vi "MAVLink Message State Machine.vi"(8 "Error In":errorcluster, 11 "Incoming Bytes":u8) -> (0 "Error Out":errorcluster, 1 "Aircraft ID":u8, 2 "Message":string, 3 "Message Complete":bool)   [LabVIEW 2014]
uses:
  CRC/MAVLink CRC v2 Check.vi
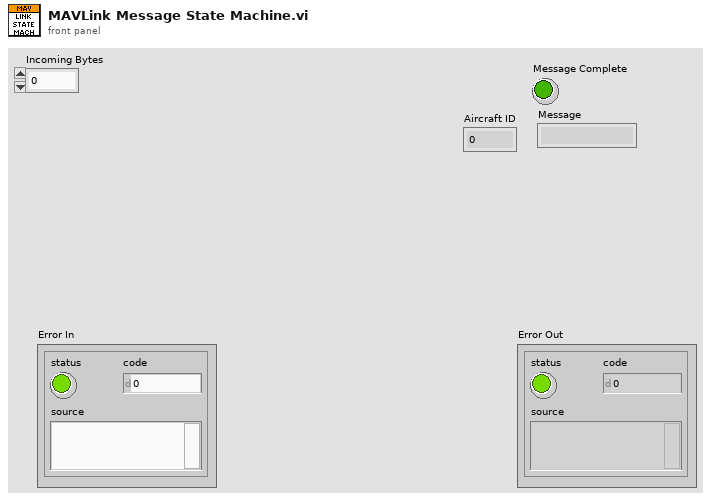
[diagram p1: front panel]
types:
  T1 = enum16{"Waiting For Start Byte", "Calculate Message Size", "Build Message"}
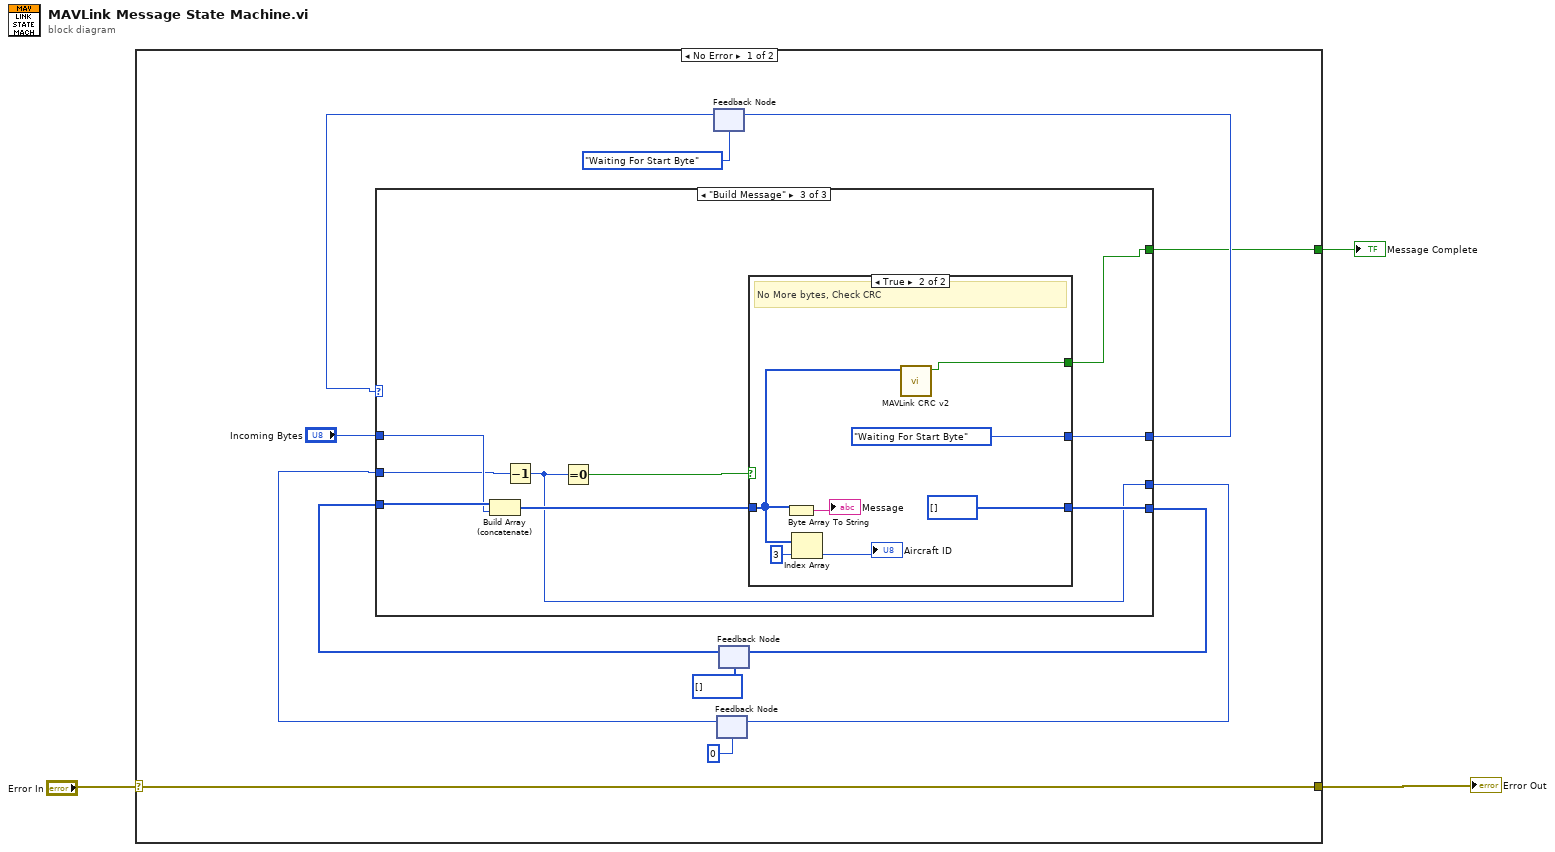
[diagram p0: block diagram]
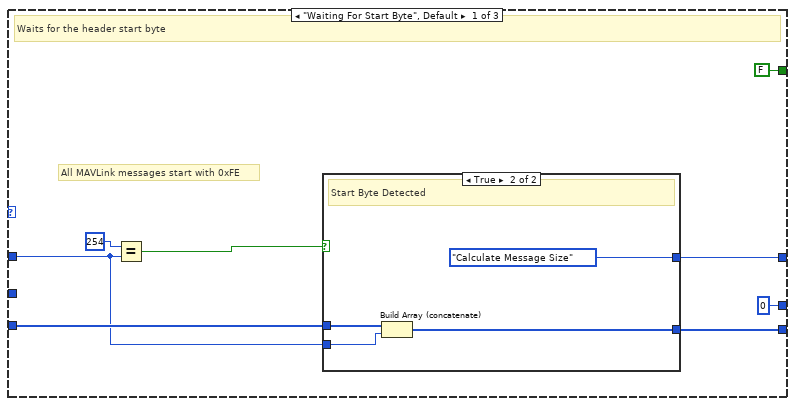
[diagram p2: hidden frame]
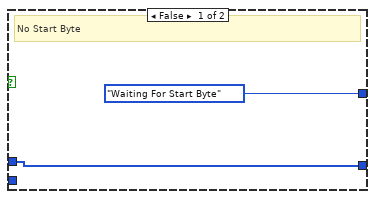
[diagram p3: hidden frame]
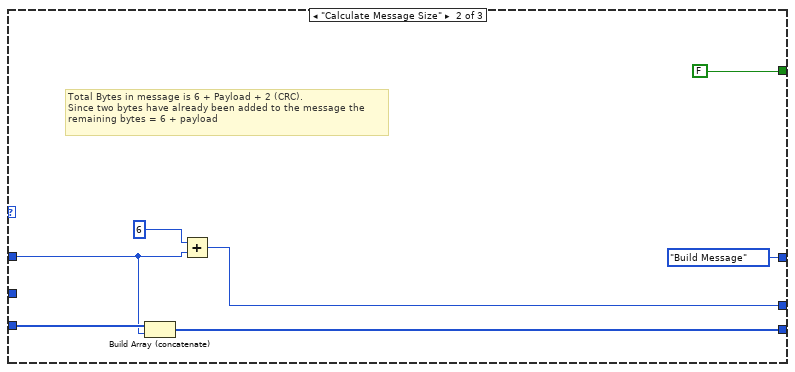
[diagram p4: hidden frame]
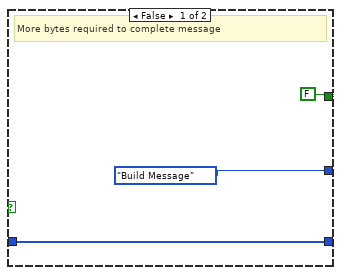
[diagram p5: hidden frame]
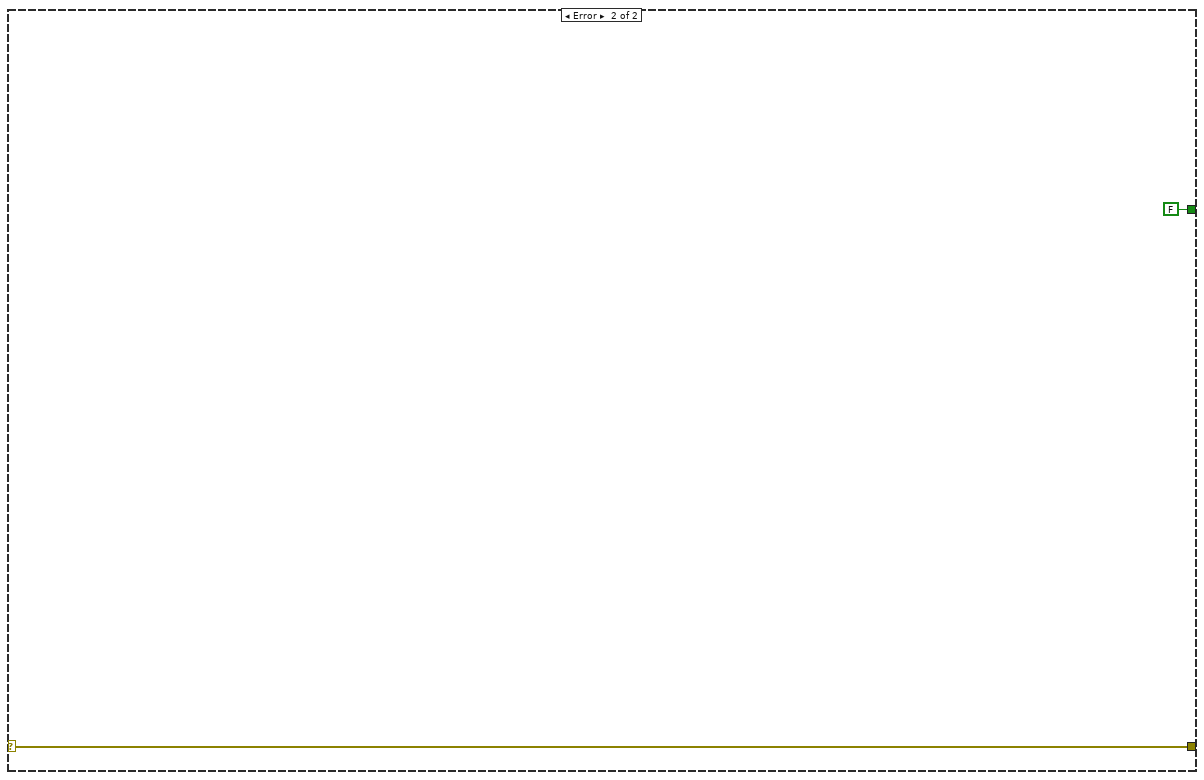
[diagram p6: hidden frame]
diagram:
  n1 = case shown="No Error" "Error In" {
    selector: "Error In" -> [w4 w57]
    tunnel: [w5 FALSE ("CRC good")] -> w3
    tunnel: [w4 w57] -> w1
    frame No Error {
      n2 = feedback #1(T1."Waiting For Start Byte" ("Message States")) -> (w14:T1)
      n3 = feedback #2(u8 0 ("x")) -> (w7:u8)
      n4 = feedback #3(u8[] []) -> (w12:u8[])
      n5 = case shown="\"Build Message\"" w14 {
        tunnel: w12 -> [w21 w34 w45]
        tunnel: "Incoming Bytes" -> [w20 w33 w44]
        tunnel: [w19 w32 w41] -> w10
        tunnel: [w18 T1."Build Message" ("Message States") w40] -> w9
        tunnel: w7 -> [_ _ w43]
        tunnel: [u8 0 w31 w39] -> w6
        tunnel: [FALSE FALSE w37] -> w5
        frame "Waiting For Start Byte", Default {
          # "All MAVLink messages start with 0xFE"
          # "Waits for the header start byte"
          n6 = Equal?(x=u8 254, y=w20) -> (x = y?=w22:bool)
          n7 = case shown="True" w22 {
            tunnel: w21 -> [w25 w29]
            tunnel: w20 -> [_ w28]
            tunnel: [w25 w27] -> w19
            tunnel: [T1."Waiting For Start Byte" ("Message States") T1."Calculate Message Size" ("Message States")] -> w18
            frame False {
              # "No Start Byte"
            }
            frame True {
              # "Start Byte Detected"
              n8 = Build Array (concatenate)(w29, w28) -> (w27:u8[])
            }
          }
        }
        frame "Calculate Message Size" {
          # "Total Bytes in message is 6 + Payload + 2 (CRC).\nSince two bytes have already been added to the message the\nremaining bytes = 6 + payload"
          n9 = Build Array (concatenate)(w34, w33) -> (w32:u8[])
          n10 = Add(x=u8 6 ("y"), y=w33) -> (x+y=w31:u8)
        }
        frame "Build Message" {
          n11 = Build Array (concatenate)(w45, w44) -> (w42:u8[])
          n12 = Decrement(x=w43) -> (x-1=w39:u8)
          n13 = Equal To 0?(x=w39) -> (x = 0?=w38:bool)
          n14 = case shown="True" w38 {
            tunnel: w42 -> [w48 w49]
            tunnel: [w48 u8[] []] -> w41
            tunnel: [T1."Build Message" ("Message States") T1."Waiting For Start Byte" ("Message States")] -> w40
            tunnel: [FALSE ("good crc") w50] -> w37
            frame False {
              # "More bytes required to complete message"
            }
            frame True {
              # "No More bytes, Check CRC"
              n15 = Byte Array To String(unsigned byte array=w49) -> (string=→"Message":string)
              n16 = Index Array(array=w49, index=3) -> (element=→"Aircraft ID":u8)
              n17 = call-poly "MAVLink CRC v2.vi"("Message"=w49) -> ("CRC good"=w50:bool)  [unwired: 10 in]
            }
          }
        }
      }
      n18 = feedback-in #1(w9) -> ()
      n19 = feedback-in #2(w6) -> ()
      n20 = feedback-in #3(w10) -> ()
    }
    frame Error {
    }
  }
  "Message Complete" <- w3
  "Error Out" <- w1
